vi "ResetDefaultValues.vi"() -> ()   [LabVIEW 2018]
panel:
  out "Slide Value":dbl
  out "Triggered":bool
  in  "Threshold":dbl
  in  "Slide":dbl(slide) scale=0.0..10.0
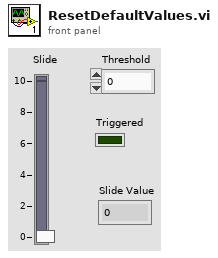
[diagram p1: front panel]
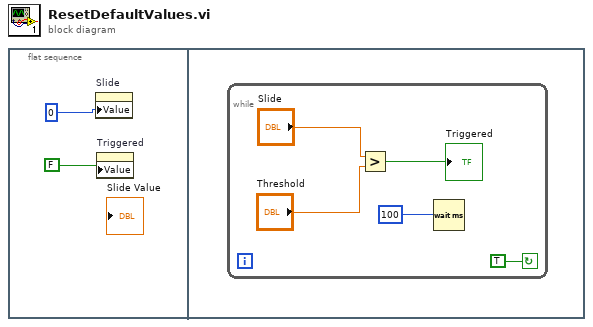
[diagram p0: block diagram]
diagram:
  n1 = flat-sequence {
    frame #0 {
      n2 = property on="Slide" class="Slide (strict)"("Value"=0) -> ()  [unwired: 2 in, 2 out]
      n3 = property on="Triggered" class="Bool (strict)"("Value"=FALSE) -> ()  [unwired: 2 in, 2 out]
    }
    frame #1 {
      n4 = while {
        stop <- TRUE continue-if-true
        n5 = Greater?(x="Slide", y="Threshold") -> (0:→"Triggered":bool)
        n6 = Wait (ms)(milliseconds to wait=100) -> ()  [unwired: 1 out]
      }
    }
  }
